vi "Wykres.vi"(9 "new element/subarray":dbl, 10 "initialized array":dbl[](array[numeric]), 11 "Y":dbl) -> (3 "output array":dbl[](array[numeric]))   [LabVIEW 2019]
panel:
  in  "index":i32
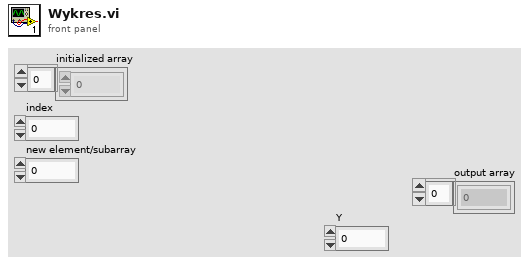
[diagram p1: front panel]
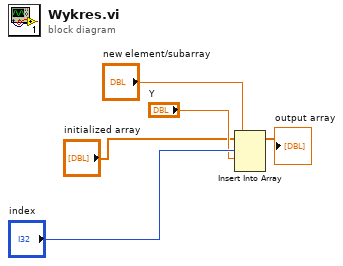
[diagram p0: block diagram]
diagram:
  n1 = Insert Into Array(array="initialized array", index="index", new element #1="Y", new element #2="new element/subarray") -> (→"output array":dbl[])
